vi "idn_action.vi"(0 "HGF_DeviceBase":refnum<class "HGF_DeviceBase.lvclass">, 5 "error in (no error)":errorcluster) -> (12 "resourceString":string, 13 "additionalInfo":string, 14 "dup HGF_DeviceBase":refnum<class "HGF_DeviceBase.lvclass">, 15 "driverRevision":string="unknown", 16 "firmwareRevision":string="unknown", 17 "vendor":string="unknown", 18 "model":string="unknown", 19 "error out":errorcluster)   [LabVIEW 2014, in "HGF_DeviceBaseClasses.lvlib" / "HGF_DeviceBase.lvclass"]
doc: "This VI queries the current instrument firmware revision and instrument driver revision.\n\nFor detailed driver information including modification history, refer to the Readme file.\n\n<b>Hint:</b> This is a dynamic dispatch VI to be implemented by child classes."
uses:
  HGF_DeviceBase.lvclass
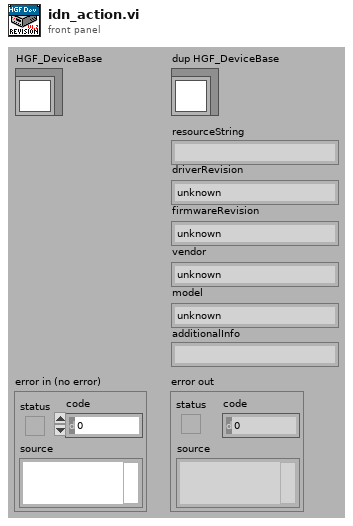
[diagram p1: front panel]
types:
  T1 = cluster{"Major":u16, "Minor":u16, "Fix":u16, "Build":u16}
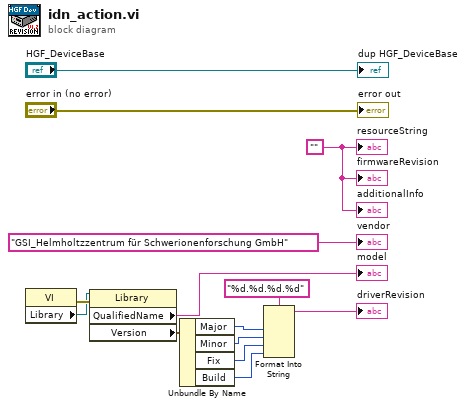
[diagram p0: block diagram]
diagram:
  w12 = ""
  n1 = property class="VI"() -> (error out=w2:errorcluster, "Library"=w1:refnum<vi>)  [unwired: 2 in, 1 out]
  n2 = property class="Library"(reference=w1, error in=w2) -> ("QualifiedName"=→"model":string, "Version"=w10:T1)  [unwired: 2 out]
  n3 = Unbundle By Name(w10) -> ("Major"=w9:u16, "Minor"=w8:u16, "Fix"=w7:u16, "Build"=w6:u16)
  n4 = Format Into String(format string="%d.%d.%d.%d", w9, w8, w7, w6) -> (resulting string=→"driverRevision":string)  [unwired: 2 in, 1 out]
  "error out" <- "error in (no error)"
  "dup HGF_DeviceBase" <- "HGF_DeviceBase"
  "firmwareRevision" <- w12
  "vendor" <- "GSI_Helmholtzzentrum für Schwerionenforschung GmbH" ("vendor")
  "resourceString" <- w12
  "additionalInfo" <- w12
